vi "Process Falling Edge.vi"(6 "edge number (1)":i32=1 min=1, 8 "error in":errorcluster, 10 "PulseAnalysis in":T1, 11 "ChannelData in":waveform(dbl)) -> (0 "error out":errorcluster, 2 "PulseAnalysis out":T1, 3 "ChannelData Out":waveform(dbl))   [LabVIEW 2019, in "Variant Parser.lvlib" / "WaveformProcessor.lvclass"]
uses:
  Library/WaveformProcessor.lvclass
  Custom Controls/Pulse Analysis.ctl
  <vilib>/measure/mascope.llb/Transition Measurements 1 chan.vi
  <vilib>/measure/NI_MAPro.lvlib
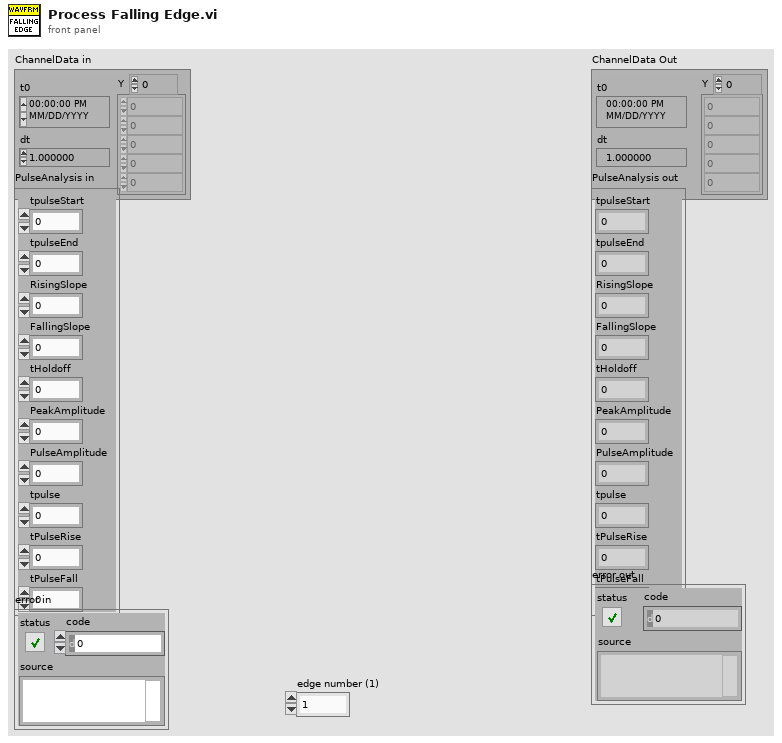
[diagram p1: front panel]
types:
  T1 = typedef "Variant Parser.lvlib/WaveformProcessor.lvclass/Pulse Analysis.ctl" = cluster{"tpulseStart":dbl, "tpulseEnd":dbl, "RisingSlope":dbl, "FallingSlope":dbl, "tHoldoff":dbl, "PeakAmplitude":dbl, "PulseAmplitude":dbl, "tpulse":dbl, "tPulseRise":dbl, "tPulseFall":dbl}
  T2 = cluster{"start time":dbl, "end time":dbl, "ref levels":cluster{"high ref level":dbl, "mid ref level":dbl, "low ref level":dbl, "ref units":u16}}
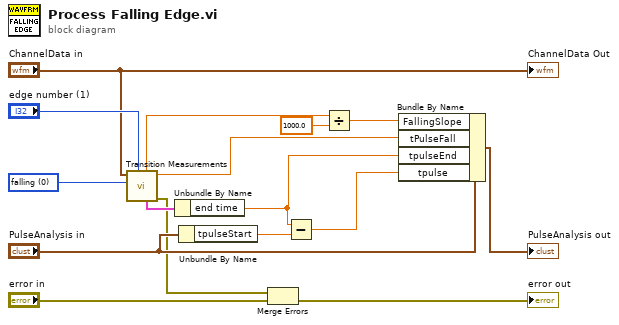
[diagram p0: block diagram]
diagram:
  w9 = u16 0 items=["falling", "rising"] ("polarity (rising)")
  n1 = call-poly <vilib>:"Transition Measurements.vi"("edge number (1)"="edge number (1)", "polarity (rising)"=w9, "signal in"="ChannelData in") -> ("error out"=w2:errorcluster, "transition duration"=w1:dbl, "measurement info"=w12:T2, "slope"=w7:dbl)  [unwired: 3 in, 2 out]
  n2 = Unbundle By Name(w12) -> ("end time"=w14:dbl)
  n3 = Unbundle By Name("PulseAnalysis in") -> ("tpulseStart"=w13:dbl)
  n4 = Merge Errors(w2, "error in") -> (→"error out":errorcluster)
  n5 = Subtract(x=w14, y=w13) -> (x-y=w15:dbl)
  n6 = Divide(x=w7, y=1000.0) -> (x/y=w11:dbl)
  n7 = Bundle By Name(cluster="PulseAnalysis in", "FallingSlope"=w11, "tPulseFall"=w1, "tpulseEnd"=w14, "tpulse"=w15) -> (→"PulseAnalysis out":T1)
  "ChannelData Out" <- "ChannelData in"
